vi "waitTarget.vi"(8 "GetPOS":refnum<vi>, 10 "Position (mm)":sgl, 11 ".NET Refnum in":refnum<k24>) -> (2 "GetPOS X (mm)":dbl format="%#_6f", 3 ".NET Refnum out":refnum<k24>)   [LabVIEW 2014]
doc: "André Romero - 2018\nandretec@ifsc.usp.br"
uses:
  C:/users-lab/Andre/GITs/andretec/Thorlabs-Vector-Move/kinesisTec/Kinesis/Thorlabs.MotionControl.TCube.DCServoCLI.dll
  Kinesis/Thorlabs.MotionControl.TCube.DCServoCLI.dll
panel:
  in  "error":dbl=0.004 format="%#_13g"
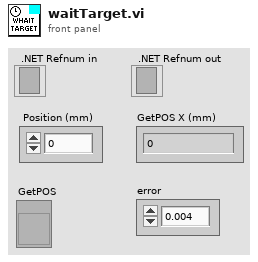
[diagram p1: front panel]
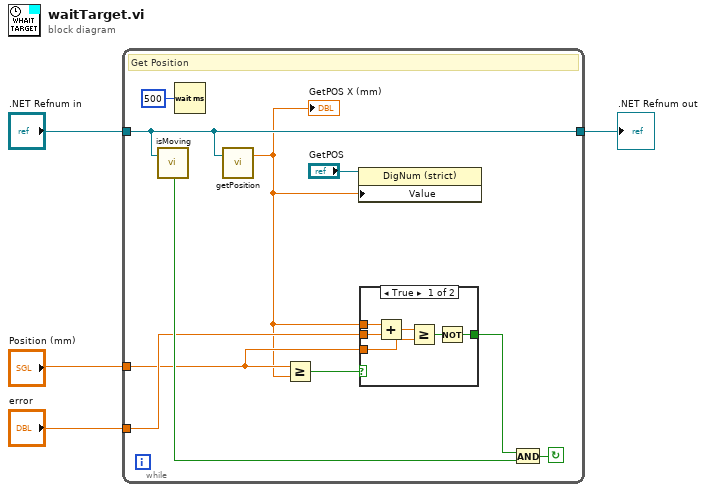
[diagram p0: block diagram]
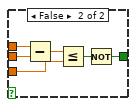
[diagram p2: hidden frame]
diagram:
  n1 = while {
    tunnel: ".NET Refnum in" -> [w14]
    tunnel: [w14] -> w3
    tunnel: "Position (mm)" -> [w7]
    tunnel: "error" -> [w8]
    stop <- w11 continue-if-true
    # "Get Position"
    n2 = call "isMoving.vi"("Device in"=w14) -> ("IsMoving"=w12:bool)  [unwired: 2 in]
    n3 = Wait (ms)(milliseconds to wait=u32 500) -> ()  [unwired: 1 out]
    n4 = call "getPosition.vi"("Device"=w14) -> ("GetPOS"=w5:dbl)  [unwired: 2 in]
    "GetPOS X (mm)" <- w5
    n5 = Greater Or Equal?(x=w7, y=w5) -> (x >= y?=w9:bool)
    n6 = property class="DigNum (strict)"(reference="GetPOS", "Value"=w5) -> ()  [unwired: 1 in, 2 out]
    n7 = case shown="True" w9 {
      tunnel: w5 -> [w20 w26]
      tunnel: w8 -> [w19 w25]
      tunnel: w7 -> [w17 w23]
      tunnel: [w15 w21] -> w6
      frame True {
        n8 = Add(x=w20, y=w19) -> (x+y=w18:dbl)
        n9 = Greater Or Equal?(x=w18, y=w17) -> (x >= y?=w16:bool)
        n10 = Not(x=w16) -> (.not. x?=w15:bool)
      }
      frame False {
        n11 = Subtract(x=w26, y=w25) -> (x-y=w24:dbl)
        n12 = Less Or Equal?(x=w24, y=w23) -> (x <= y?=w22:bool)
        n13 = Not(x=w22) -> (.not. x?=w21:bool)
      }
    }
    n14 = And(x=w6, y=w12) -> (x .and. y?=w11:bool)
  }
  ".NET Refnum out" <- w3
